vi "Update_WF.vi"(8 "entrée d'erreur (pas d'erreur)":errorcluster) -> (0 "sortie d'erreur":errorcluster, 1 "Waveform Graph 2":waveform(dbl)[](array[waveform]), 2 "Waveform Graph":waveform(dbl)[](array[waveform]), 3 "DO Master":digitalwaveform[](graph))   [LabVIEW 2026]
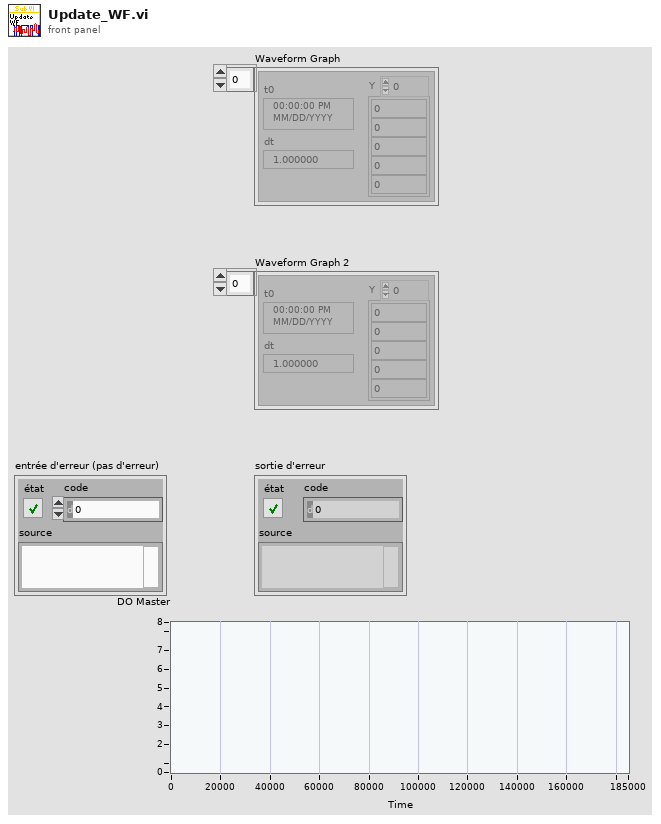
[diagram p1: front panel]
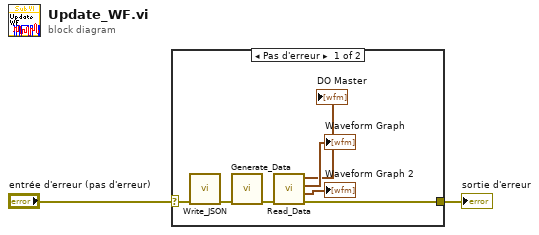
[diagram p0: block diagram]
diagram:
  n1 = case shown="Pas d'erreur" "entrée d'erreur (pas d'erreur)" {
    selector: "entrée d'erreur (pas d'erreur)" -> [w6 w10]
    tunnel: [w9 w10] -> w2
    frame No Error {
      n2 = call "Write_JSON.vi"("error in"=w6) -> ("error out"=w7:errorcluster)  [unwired: 8 in]
      n3 = call "Generate_Data.vi"("error in"=w7) -> ("error out"=w8:errorcluster)  [unwired: 10 in]
      n4 = call "Read_Data.vi"("error in"=w8) -> ("error out"=w9:errorcluster, "AO Slave"=→"Waveform Graph 2":waveform(dbl)[], "AO Master"=→"Waveform Graph":waveform(dbl)[], "DO Master"=→"DO Master":digitalwaveform[])  [unwired: 7 in]
    }
    frame Error {
    }
  }
  "sortie d'erreur" <- w2
